vi "AvoidancePolygon.vi"(1 "Arm Pass Through Params":T1, 2 "RobotConfig":T2={"Motors"={"DriveRightPrimary"={"CAN Address"=3, "Invert"=FALSE, "InvertSensor"=FALSE, "Unit Conversion Factor"=0.0, "Brake Mode"=enum."Override to Brake", "Reverse Limt Switch Mode"=enum."Normally Closed", "Forward Limt Swith Mode"=enum."Normally Closed", "PWM Channel"=enum."Invalid", "Motor Controller Type"=enum."Talon SRX", "Peak Current (A)"=0, "Continuous Current (A)"=0, "Peak Duration (ms)"=0, "Current Limit Enable"=FALSE}, "DriveRightSecondary"={"CAN Address"=2, "Invert"=FALSE, "InvertSensor"=FALSE, "Unit Conversion Factor"=0.0, "Brake Mode"=enum."Override to Brake", "Reverse Limt Switch Mode"=enum."Normally Closed", "Forward Limt Swith Mode"=enum."Normally Closed", "PWM Channel"=enum."Invalid", "Motor Controller Type"=enum."Talon SRX", "Peak Current (A)"=0, "Continuous Current (A)"=0, "Peak Duration (ms)"=0, "Current Limit Enable"=FALSE}, "DriveLeftPrimary"={"CAN Address"=1, "Invert"=FALSE, "InvertSensor"=FALSE, "Unit Conversion Factor"=0.0, "Brake Mode"=enum."Override to Brake", "Reverse Limt Switch Mode"=enum."Normally Closed", "Forward Limt Swith Mode"=enum."Normally Closed", "PWM Channel"=enum."Invalid", "Motor Controller Type"=enum."Talon SRX", "Peak Current (A)"=0, "Continuous Current (A)"=0, "Peak Duration (ms)"=0, "Current Limit Enable"=FALSE}, "DriveLeftSecondary"={"CAN Address"=4, "Invert"=FALSE, "InvertSensor"=FALSE, "Unit Conversion Factor"=0.0, "Brake Mode"=enum."Override to Brake", "Reverse Limt Switch Mode"=enum."Normally Closed", "Forward Limt Swith Mode"=enum."Normally Closed", "PWM Channel"=enum."Invalid", "Motor Controller Type"=enum."Talon SRX", "Peak Current (A)"=0, "Continuous Current (A)"=0, "Peak Duration (ms)"=0, "Current Limit Enable"=FALSE}, "RearClimb"={"CAN Address"=8, "Invert"=FALSE, "InvertSensor"=FALSE, "Unit Conversion Factor"=0.0, "Brake Mode"=enum."Override to Brake", "Reverse Limt Switch Mode"=enum."Normally Closed", "Forward Limt Swith Mode"=enum."Normally Closed", "PWM Channel"=enum."Invalid", "Motor Controller Type"=enum."Talon SRX", "Peak Current (A)"=0, "Continuous Current (A)"=0, "Peak Duration (ms)"=0, "Current Limit Enable"=FALSE}, "Front Climb"={"CAN Address"=7, "Invert"=FALSE, "InvertSensor"=FALSE, "Unit Conversion Factor"=0.0, "Brake Mode"=enum."Override to Brake", "Reverse Limt Switch Mode"=enum."Normally Closed", "Forward Limt Swith Mode"=enum."Normally Closed", "PWM Channel"=enum."Invalid", "Motor Controller Type"=enum."Talon SRX", "Peak Current (A)"=0, "Continuous Current (A)"=0, "Peak Duration (ms)"=0, "Current Limit Enable"=FALSE}, "Climb Drive"={"CAN Address"=5, "Invert"=FALSE, "InvertSensor"=FALSE, "Unit Conversion Factor"=0.0, "Brake Mode"=enum."Override to Brake", "Reverse Limt Switch Mode"=enum."Normally Closed", "Forward Limt Swith Mode"=enum."Normally Closed", "PWM Channel"=enum."Invalid", "Motor Controller Type"=enum."Talon SRX", "Peak Current (A)"=0, "Continuous Current (A)"=0, "Peak Duration (ms)"=0, "Current Limit Enable"=FALSE}, "Shoulder1"={"CAN Address"=6, "Invert"=FALSE, "InvertSensor"=FALSE, "Unit Conversion Factor"=0.0, "Brake Mode"=enum."Override to Brake", "Reverse Limt Switch Mode"=enum."Normally Closed", "Forward Limt Swith Mode"=enum."Normally Closed", "PWM Channel"=enum."Invalid", "Motor Controller Type"=enum."Talon SRX", "Peak Current (A)"=0, "Continuous Current (A)"=0, "Peak Duration (ms)"=0, "Current Limit Enable"=FALSE}, "Shoulder2"={"CAN Address"=9, "Invert"=FALSE, "InvertSensor"=FALSE, "Unit Conversion Factor"=0.0, "Brake Mode"=enum."Override to Brake", "Reverse Limt Switch Mode"=enum."Normally Closed", "Forward Limt Swith Mode"=enum."Normally Closed", "PWM Channel"=enum."Invalid", "Motor Controller Type"=enum."Talon SRX", "Peak Current (A)"=0, "Continuous Current (A)"=0, "Peak Duration (ms)"=0, "Current Limit Enable"=FALSE}, "Wrist"={"CAN Address"=10, "Invert"=FALSE, "InvertSensor"=FALSE, "Unit Conversion Factor"=0.0, "Brake Mode"=enum."Override to Brake", "Reverse Limt Switch Mode"=enum."Disabled", "Forward Limt Swith Mode"=enum."Disabled", "PWM Channel"=enum."Invalid", "Motor Controller Type"=enum."Talon SRX", "Peak Current (A)"=0, "Continuous Current (A)"=0, "Peak Duration (ms)"=0, "Current Limit Enable"=FALSE}, "Extension"={"CAN Address"=11, "Invert"=FALSE, "InvertSensor"=FALSE, "Unit Conversion Factor"=0.0, "Brake Mode"=enum."Override to Brake", "Reverse Limt Switch Mode"=enum."Disabled", "Forward Limt Swith Mode"=enum."Disabled", "PWM Channel"=enum."Invalid", "Motor Controller Type"=enum."Talon SRX", "Peak Current (A)"=0, "Continuous Current (A)"=0, "Peak Duration (ms)"=0, "Current Limit Enable"=FALSE}, "CargoIntake"={"CAN Address"=0, "Invert"=FALSE, "InvertSensor"=FALSE, "Unit Conversion Factor"=1.0, "Brake Mode"=enum."Override to Brake", "Reverse Limt Switch Mode"=enum."Disabled", "Forward Limt Swith Mode"=enum."Normally Open", "PWM Channel"=enum."PWM 8", "Motor Controller Type"=enum."Talon SR", "Peak Current (A)"=0, "Continuous Current (A)"=0, "Peak Duration (ms)"=0, "Current Limit Enable"=FALSE}, "Intake2"={"CAN Address"=10, "Invert"=FALSE, "InvertSensor"=TRUE, "Unit Conversion Factor"=0.0, "Brake Mode"=enum."Override to Brake", "Reverse Limt Switch Mode"=enum."Normally Open", "Forward Limt Swith Mode"=enum."Normally Open", "PWM Channel"=enum."PWM 0", "Motor Controller Type"=enum."Disabled", "Peak Current (A)"=0, "Continuous Current (A)"=0, "Peak Duration (ms)"=0, "Current Limit Enable"=FALSE}}, "Sensors"={"IMU"={"Yaw Axis"=enum."Z", "SPI Bus"=enum."SPI MXP", "AHRS Algorithm"=enum."Complementary", "Calibration Time (s)"=3.0, "Calibrate On Open"=TRUE}, "HomingButton"={"DIOChannel"=enum."DIO 0", "Active Low"=FALSE}, "HomingLED_Green"={"DIOChannel"=enum."DIO 0", "Active Low"=FALSE}, "HomingLED_Yellow"={"DIOChannel"=enum."DIO 0", "Active Low"=FALSE}, "HomingLED_Red"={"DIOChannel"=enum."DIO 0", "Active Low"=FALSE}}, "PID"={"FrontClimb"={"P"=0.0, "I"=0.0, "D"=0.0, "F"=0.0, "IZone"=0.0}, "RearClimb"={"P"=0.0, "I"=0.0, "D"=0.0, "F"=0.0, "IZone"=0.0}, "ArmShoulder"={"P"=0.0, "I"=0.0, "D"=0.0, "F"=0.0, "IZone"=0.0}, "ArmExtend"={"P"=0.0, "I"=0.0, "D"=0.0, "F"=0.0, "IZone"=0.0}, "ArmWrist"={"P"=0.0, "I"=0.0, "D"=0.0, "F"=0.0, "IZone"=0.0}}, "Solenoids"={" Shifter"={"SolenoidChannel"=enum."Solenoid 3", "Invert"=FALSE}, "Hatch Grip"={"SolenoidChannel"=enum."Solenoid 0", "Invert"=FALSE}, "Hatch Extend"={"SolenoidChannel"=enum."Solenoid 1", "Invert"=FALSE}, "Manipulator Slide"={"SolenoidChannel"=enum."Solenoid 2", "Invert"=FALSE}, "Hatch Floor Intake"={"SolenoidChannel"=enum."Solenoid 0", "Invert"=FALSE}}, "Enable Compressor"=TRUE, "MotionMagic"={"FrontClimbExtend"={"CruiseVelocity"=0, "Acceleration"=0}, "RearClimbExtend"={"CruiseVelocity"=0, "Acceleration"=0}, "FrontClimbRetract"={"CruiseVelocity"=0, "Acceleration"=0}, "RearClimbRetract"={"CruiseVelocity"=0, "Acceleration"=0}}, "RobotDimensions"={"Length (in)"=0.0, "Shoulder Height (in)"=0.0, "Frame Height (in)"=0.0, "Arm Center to Front of Robot (in)"=0.0, "Arm Min Extension (in)"=0.0, "Arm Max Extension (in)"=0.0, "Cargo Intake Loop Length (in)"=0.0, "Cargo Intake Loop Width (in)"=0.0, "Cargo Intake Loop Offset (in)"=0.0, "Cargo Intake Loop Angle (rad)"=0.0}, "Arm Home Position"={"Radius (in)"=0.0, "ShoulderAngle (rad)"=0.0, "WristAngle (rad)"=0.0}, "Climb Home Position"={"Back Climb"=0.0, "Front Climb"=0.0}, "Climb Positions"={"Retract"=0.0, "Level 2"=0.0, "Level 3"=0.0}}) -> (0 "Polygon":T19)   [LabVIEW 2018]
uses:
  ArgosLib/Path Planning/TypeDefs/Polygon2D.ctl
  ArgosLib/Path Planning/TypeDefs/Point2D.ctl
  TypeDefs/ConfigComponents/Config_Robot.ctl
  ArgosLib/Config/ConfigComponents/TypeDefs/Config_Motor.ctl
  <vilib>/Rock Robotics/WPI/ThirdParty/Phoenix-LabVIEW/Motor Controller/Controls/CTRE_Phoenix_MotorControl_NeutralMode.ctl
  <vilib>/Rock Robotics/WPI/ThirdParty/Phoenix-LabVIEW/Motor Controller/Controls/CTRE_Phoenix_MotorControl_LimitSwitchNormal.ctl
  <vilib>/Rock Robotics/SystemInterfaces/DIO/FPGA_DIOPWMChannel.ctl
  ArgosLib/Config/ConfigComponents/TypeDefs/Config_MotorCtrlType.ctl
  ArgosLib/Config/ConfigComponents/TypeDefs/Config_IMU.ctl
  <vilib>/Rock Robotics/SystemInterfaces/spilib/spi_bus.ctl
  ArgosLib/Config/ConfigComponents/TypeDefs/Config_DigitalIO.ctl
  <vilib>/Rock Robotics/SystemInterfaces/DIO/FPGA_DIOChannel.ctl
  ArgosLib/Config/ConfigComponents/TypeDefs/Config_PIDParams.ctl
  ArgosLib/Config/ConfigComponents/TypeDefs/Config_SingleSolenoid.ctl
  <vilib>/Rock Robotics/WPI/Solenoid/WPI_SolenoidChannel.ctl
  ArgosLib/Config/ConfigComponents/TypeDefs/Config_MotionMagicParams.ctl
  TypeDefs/ConfigComponents/Config_Dimensions.ctl
  TypeDefs/ArmCoordinate.ctl
  Climber/TypeDefs/ClimberPositionHeights.ctl
  TypeDefs/ArmPassThroughParams.ctl
  ArgosLib/ArgosLib.lvlib
panel:
  in  "Max Height (in)":dbl=90.0
  in  "Max Frame Extension (in)":dbl=30.0
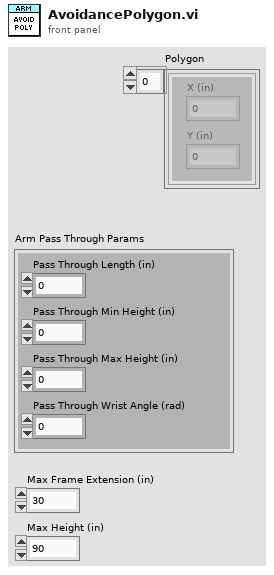
[diagram p1: front panel]
types:
  T1 = typedef "ArmPassThroughParams.ctl" = cluster{"Pass Through Length (in)":dbl, "Pass Through Min Height (in)":dbl, "Pass Through Max Height (in)":dbl, "Pass Through Wrist Angle (rad)":dbl}
  T2 = typedef "Config_Robot.ctl" = cluster{"Motors":cluster{"DriveRightPrimary":T3, "DriveRightSecondary":T3, "DriveLeftPrimary":T3, "DriveLeftSecondary":T3, "RearClimb":T3, "Front Climb":T3, "Climb Drive":T3, "Shoulder1":T3, "Shoulder2":T3, "Wrist":T3, "Extension":T3, "CargoIntake":T3, "Intake2":T3}, "Sensors":cluster{"IMU":T8, "HomingButton":T10, "HomingLED_Green":T10, "HomingLED_Yellow":T10, "HomingLED_Red":T10}, "PID":cluster{"FrontClimb":T12, "RearClimb":T12, "ArmShoulder":T12, "ArmExtend":T12, "ArmWrist":T12}, "Solenoids":cluster{" Shifter":T13, "Hatch Grip":T13, "Hatch Extend":T13, "Manipulator Slide":T13, "Hatch Floor Intake":T13}, "Enable Compressor":bool, "MotionMagic":cluster{"FrontClimbExtend":T15, "RearClimbExtend":T15, "FrontClimbRetract":T15, "RearClimbRetract":T15}, "RobotDimensions":T16, "Arm Home Position":T17, "Climb Home Position":cluster{"Back Climb":dbl, "Front Climb":dbl}, "Climb Positions":T18}
  T3 = typedef "ArgosLib.lvlib/Config_Motor.ctl" = cluster{"CAN Address":u8, "Invert":bool, "InvertSensor":bool, "Unit Conversion Factor":dbl, "Brake Mode":T4, "Reverse Limt Switch Mode":T5, "Forward Limt Swith Mode":T5, "PWM Channel":T6, "Motor Controller Type":T7, "Peak Current (A)":i32, "Continuous Current (A)":i32, "Peak Duration (ms)":i32, "Current Limit Enable":bool}
  T4 = typedef "CTRE_Phoenix_MotorControl_NeutralMode.ctl" = enum8{"EEPROMSetting", "Override to Coast", "Override to Brake"}
  T5 = typedef "CTRE_Phoenix_MotorControl_LimitSwitchNormal.ctl" = enum16{"Normally Open", "Normally Closed", "Disabled"}
  T6 = typedef "FPGA_DIOPWMChannel.ctl" = enum8{"PWM 0", "PWM 1", "PWM 2", "PWM 3", "PWM 4", "PWM 5", "PWM 6", "PWM 7", "PWM 8", "PWM 9", "PWM MXP 0", "PWM MXP 1", "PWM MXP 2", "PWM MXP 3", "PWM MXP 4", "PWM MXP 5", "PWM MXP 6", "PWM MXP 7", "PWM MXP 8", "PWM MXP 9", "Invalid"}
  T7 = typedef "ArgosLib.lvlib/Config_MotorCtrlType.ctl" = enum16{"Disabled", "Talon SRX", "Talon SR", "Venom"}
  T8 = typedef "ArgosLib.lvlib/Config_IMU.ctl" = cluster{"Yaw Axis":enum16{"X", "Y", "Z"}, "SPI Bus":T9, "AHRS Algorithm":enum16{"Complementary", "Madgwick"}, "Calibration Time (s)":dbl, "Calibrate On Open":bool}
  T9 = typedef "spi_bus.ctl" = enum16{"SPI On-Board, CS0", "SPI On-Board, CS1", "SPI On-Board, CS2", "SPI On-Board, CS3", "SPI MXP", "Invalid"}
  T10 = typedef "ArgosLib.lvlib/Config_DigitalIO.ctl" = cluster{"DIOChannel":T11, "Active Low":bool}
  T11 = typedef "FPGA_DIOChannel.ctl" = enum8{"DIO 0", "DIO 1", "DIO 2", "DIO 3", "DIO 4", "DIO 5", "DIO 6", "DIO 7", "DIO 8", "DIO 9", "DIO MXP 0", "DIO MXP 1", "DIO MXP 2", "DIO MXP 3", "DIO MXP 4", "DIO MXP 5", "DIO MXP 6", "DIO MXP 7", "DIO MXP 8", "DIO MXP 9", "DIO MXP 10", "DIO MXP 11", "DIO MXP 12", "DIO MXP 13", "DIO MXP 14", "DIO MXP 15", "SPI Port CS1", "SPI Port CS2", "SPI Port CS3", "SPI Port MISO", "SPI Port MOSI", "Invalid"}
  T12 = typedef "ArgosLib.lvlib/Config_PIDParams.ctl" = cluster{"P":dbl, "I":dbl, "D":dbl, "F":dbl, "IZone":dbl}
  T13 = typedef "ArgosLib.lvlib/Config_SingleSolenoid.ctl" = cluster{"SolenoidChannel":T14, "Invert":bool}
  T14 = typedef "WPI_SolenoidChannel.ctl" = enum8{"Solenoid 0", "Solenoid 1", "Solenoid 2", "Solenoid 3", "Solenoid 4", "Solenoid 5", "Solenoid 6", "Solenoid 7", "Invalid"}
  T15 = typedef "Config_MotionMagicParams.ctl" = cluster{"CruiseVelocity":i32, "Acceleration":i32}
  T16 = typedef "Config_Dimensions.ctl" = cluster{"Length (in)":dbl, "Shoulder Height (in)":dbl, "Frame Height (in)":dbl, "Arm Center to Front of Robot (in)":dbl, "Arm Min Extension (in)":dbl, "Arm Max Extension (in)":dbl, "Cargo Intake Loop Length (in)":dbl, "Cargo Intake Loop Width (in)":dbl, "Cargo Intake Loop Offset (in)":dbl, "Cargo Intake Loop Angle (rad)":dbl}
  T17 = typedef "ArmCoordinate.ctl" = cluster{"Radius (in)":dbl, "ShoulderAngle (rad)":dbl, "WristAngle (rad)":dbl}
  T18 = typedef "ClimberPositionHeights.ctl" = cluster{"Retract":dbl, "Level 2":dbl, "Level 3":dbl}
  T19 = typedef "ArgosLib.lvlib/Polygon2D.ctl" = T20[]
  T20 = typedef "ArgosLib.lvlib/Point2D.ctl" = cluster{"X (in)":dbl, "Y (in)":dbl}
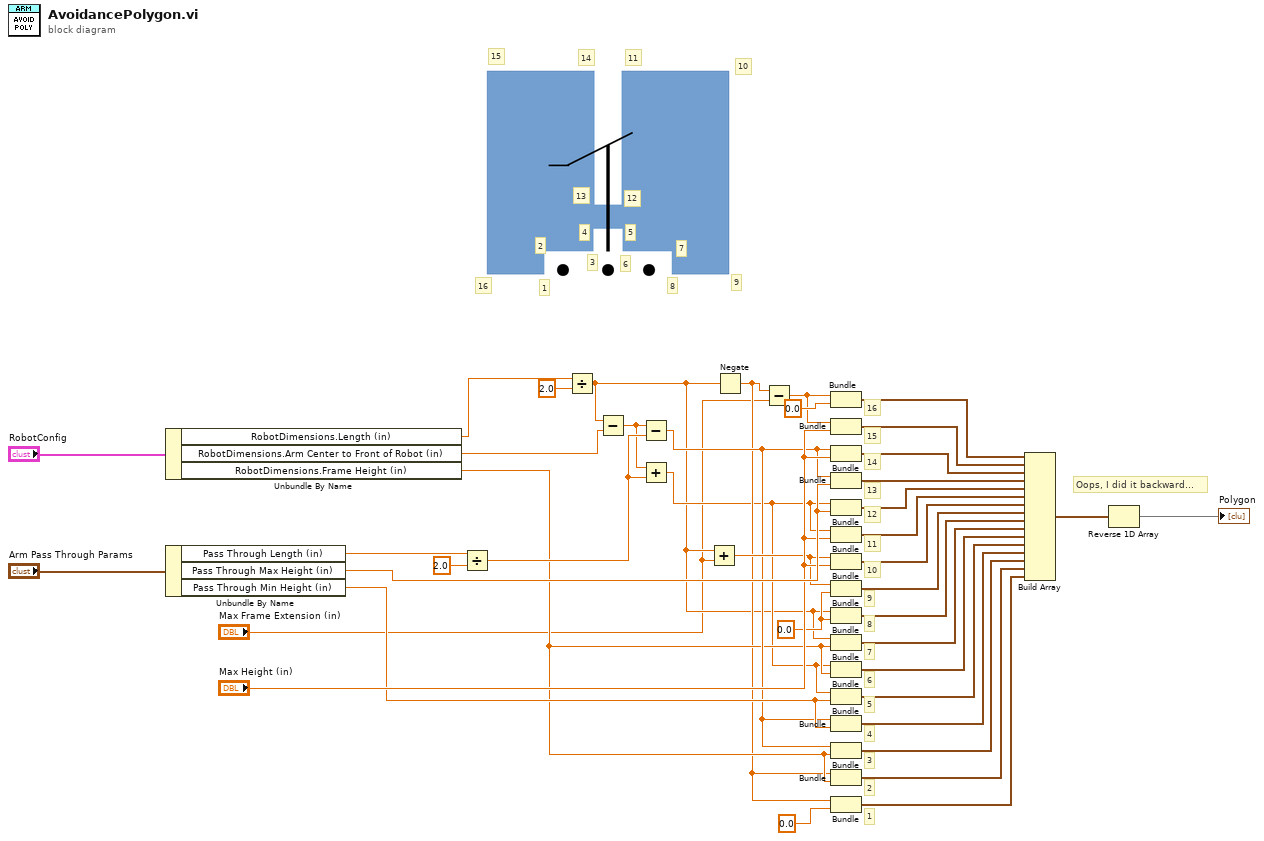
[diagram p0: block diagram]
diagram:
  w24 = 0.0 ("y")
  # "16"
  # "15"
  # "14"
  # "13"
  # "12"
  # "11"
  # "10"
  # "9"
  # "8"
  # "7"
  # "6"
  # "5"
  # "4"
  # "3"
  # "2"
  # "1"
  # "Oops, I did it backward..."
  # "15"
  # "14"
  # "13"
  # "12"
  # "11"
  # "10"
  # "9"
  # "8"
  # "7"
  # "6"
  # "5"
  # "4"
  # "3"
  # "2"
  # "1"
  # "16"
  n1 = Unbundle By Name("RobotConfig") -> ("RobotDimensions.Length (in)"=w40:dbl, "RobotDimensions.Arm Center to Front of Robot (in)"=w32:dbl, "RobotDimensions.Frame Height (in)"=w20:dbl)
  n2 = Unbundle By Name("Arm Pass Through Params") -> ("Pass Through Length (in)"=w31:dbl, "Pass Through Max Height (in)"=w27:dbl, "Pass Through Min Height (in)"=w22:dbl)
  n3 = Divide(x=w31, y=2.0) -> (x/y=w25:dbl)
  n4 = Divide(x=w40, y=2.0) -> (x/y=w2:dbl)
  n5 = Subtract(x=w2, y=w32) -> (x-y=w4:dbl)
  n6 = Subtract(x=w4, y=w25) -> (x-y=w21:dbl)
  n7 = Add(x=w4, y=w25) -> (x+y=w3:dbl)
  n8 = Add(x=w2, y="Max Frame Extension (in)") -> (x+y=w23:dbl)
  n9 = Negate(x=w2) -> (-x=w19:dbl)
  n10 = Subtract(x=w19, y="Max Frame Extension (in)") -> (x-y=w35:dbl)
  n11 = Bundle(w35, "y"=0.0) -> (w37:cluster{dbl, "y":dbl})  [unwired: 1 in]
  n12 = Bundle(w35, "Max Height (in)"="Max Height (in)") -> (w34:cluster{dbl, "Max Height (in)":dbl})  [unwired: 1 in]
  n13 = Bundle(w21, "Max Height (in)"="Max Height (in)") -> (w29:cluster{dbl, "Max Height (in)":dbl})  [unwired: 1 in]
  n14 = Bundle(w21, "Pass Through Max Height (in)"=w27) -> (w28:cluster{dbl, "Pass Through Max Height (in)":dbl})  [unwired: 1 in]
  n15 = Bundle(w3, "Pass Through Max Height (in)"=w27) -> (w17:cluster{dbl, "Pass Through Max Height (in)":dbl})  [unwired: 1 in]
  n16 = Bundle(w3, "Max Height (in)"="Max Height (in)") -> (w16:cluster{dbl, "Max Height (in)":dbl})  [unwired: 1 in]
  n17 = Bundle(w23, "Max Height (in)"="Max Height (in)") -> (w15:cluster{dbl, "Max Height (in)":dbl})  [unwired: 1 in]
  n18 = Bundle(w23, "y"=w24) -> (w14:cluster{dbl, "y":dbl})  [unwired: 1 in]
  n19 = Bundle(w2, "y"=w24) -> (w13:cluster{dbl, "y":dbl})  [unwired: 1 in]
  n20 = Bundle(w2, "Frame Height (in)"=w20) -> (w12:cluster{dbl, "Frame Height (in)":dbl})  [unwired: 1 in]
  n21 = Bundle(w3, "Frame Height (in)"=w20) -> (w11:cluster{dbl, "Frame Height (in)":dbl})  [unwired: 1 in]
  n22 = Bundle(w3, "Pass Through Min Height (in)"=w22) -> (w10:cluster{dbl, "Pass Through Min Height (in)":dbl})  [unwired: 1 in]
  n23 = Bundle(w21, "Pass Through Min Height (in)"=w22) -> (w9:cluster{dbl, "Pass Through Min Height (in)":dbl})  [unwired: 1 in]
  n24 = Bundle(w21, "Frame Height (in)"=w20) -> (w8:cluster{dbl, "Frame Height (in)":dbl})  [unwired: 1 in]
  n25 = Bundle(w19, "Frame Height (in)"=w20) -> (w7:cluster{dbl, "Frame Height (in)":dbl})  [unwired: 1 in]
  n26 = Bundle(w19, "y"=0.0) -> (w6:cluster{dbl, "y":dbl})  [unwired: 1 in]
  n27 = Build Array(w37, w34, w29, w28, w17, w16, w15, w14, w13, w12, w11, w10, w9, w8, w7, w6) -> (w36:cluster{dbl, "y":dbl}[])
  n28 = Reverse 1D Array(array=w36) -> (reversed array=→"Polygon":cluster{dbl, "y":dbl}[])
